vi "LAC Cmd080R_Sys Info.vi"(7 "timeout(ms)":u32, 8 "error in":errorcluster, 11 "VISA name in":refnum<visa-resource-name>) -> (0 "error out":errorcluster, 1 "readout":string, 3 "VISA name out":refnum<visa-resource-name>)   [LabVIEW 8.6]
panel:
  # "readout items\n*1: IPU model name\n*2: IPU serial number\n*3: IPU version\n*4: IPU MAC address\n*5: IPU manufactured date (yyyymmdd)\n*6: Sensor head model name\n*7: Sensor head serial number\n*8: Sensor head version\n*9: Sensor head manufactured date (yyyymmdd)"
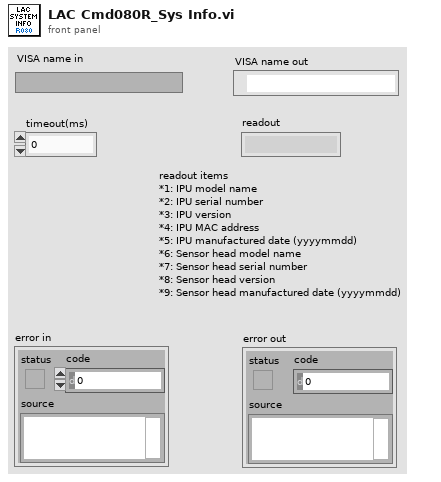
[diagram p1: front panel]
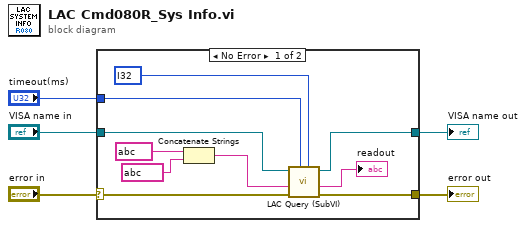
[diagram p0: block diagram]
diagram:
  n1 = case shown="No Error" "error in" {
    selector: "error in" -> [w11 w17]
    tunnel: "VISA name in" -> [w13 w16]
    tunnel: [w15 w16] -> w4
    tunnel: [w14 w17] -> w3
    tunnel: "timeout(ms)" -> [w12 _]
    frame #0 {
      n2 = Concatenate Strings(string ? ("string"), string ? ("write buffer")) -> (w9:string)
      n3 = call "LAC Query (SubVI).vi"("interval(ms)"=i32 ?, "timeout(ms)"=w12, "error in"=w11, "Command"=w9, "VISA name in"=w13) -> ("error out"=w14:errorcluster, "read buffer"=→"readout":string, "VISA name out"=w15:refnum<visa-resource-name>)  [unwired: 4 in]
    }
    frame #1 {
    }
  }
  "VISA name out" <- w4
  "error out" <- w3
